vi "Labview2Mysql.vi"() -> ()   [LabVIEW 2019]
panel:
  out "concatenated string":string
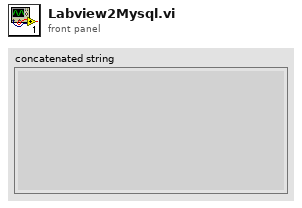
[diagram p1: front panel]
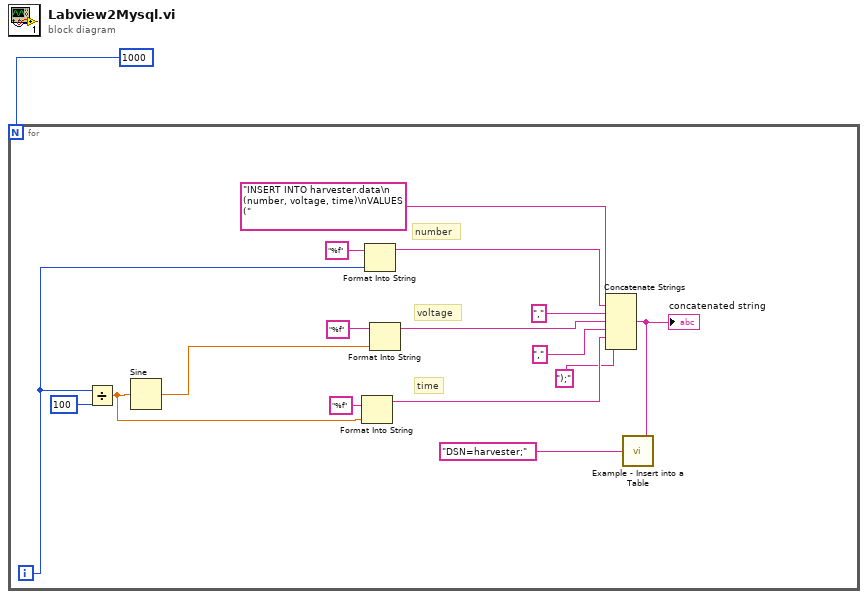
[diagram p0: block diagram]
diagram:
  n1 = for {
    N: 1000 -> [_]
    i -> [w5]
    # "time"
    # "voltage"
    # "number"
    n2 = Divide(x=w5, y=100) -> (x/y=w2:dbl)
    n3 = Sine(x=w2) -> (sin(x)=w3:dbl)
    n4 = Format Into String(format string="%f", w2) -> (resulting string=w10:string)  [unwired: 2 in, 1 out]
    n5 = Format Into String(format string="%f", w5) -> (resulting string=w14:string)  [unwired: 2 in, 1 out]
    n6 = Format Into String(format string="%f", w3) -> (resulting string=w12:string)  [unwired: 2 in, 1 out]
    n7 = Concatenate Strings("INSERT INTO harvester.data\n (number, voltage, time)\nVALUES (", w14, "," ("string"), w12, "," ("string"), w10, ");" ("string")) -> (w6:string)
    "concatenated string" <- w6
    n8 = call "Example - Insert into a Table.vi"("Command Text"=w6, "ConnectionString"="DSN=harvester;" ("Command Text")) -> ()
  }
